vi "CoMP-S Mechanism - ZeroCommnandProtection.vi"(8 "error in (no error)":errorcluster, 11 "Arg 1":sgl) -> (0 "error out":errorcluster)   [LabVIEW 2014]
doc: "Create error code and message if input value is zero"
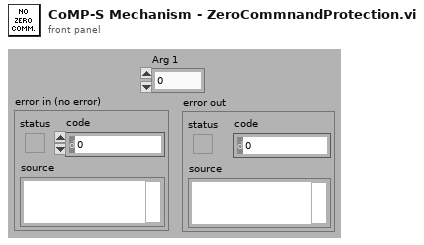
[diagram p1: front panel]
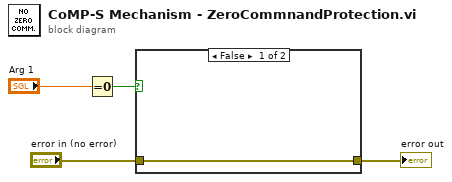
[diagram p0: block diagram]
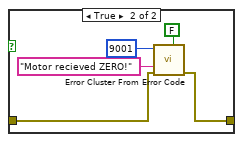
[diagram p2: hidden frame]
diagram:
  n1 = Equal To 0?(x="Arg 1") -> (x = 0?=w3:bool)
  n2 = case shown="False" w3 {
    tunnel: "error in (no error)" -> [w5 w7]
    tunnel: [w5 w6] -> w1
    frame False {
    }
    frame True {
      n3 = call <vilib>:"Error Cluster From Error Code.vi"("is warning? (False)"=FALSE, "error in (no error)"=w7, "error message (\"\")"="Motor recieved ZERO!" ("error message (\"\")"), "error code (0)"=9001) -> ("error out"=w6:errorcluster)  [unwired: 5 in]
    }
  }
  "error out" <- w1
